vi "close vi.vi"(8 "error in":errorcluster, 11 "vi id":string) -> (0 "error out":errorcluster)   [LabVIEW 2020]
doc: "Closes a currently open VI frontpanel window. If VI was not saved it will be deleted by this."
uses:
  G-AI Core/G-AI Core.lvlib
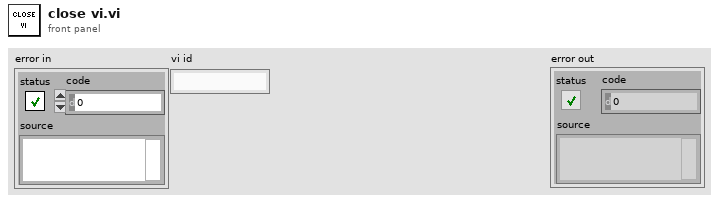
[diagram p1: front panel]
types:
  T1 = enum32{"Invalid", "Standard", "Closed", "Hidden", "Minimized", "Maximized"}
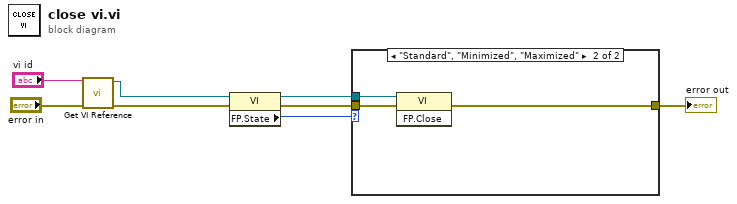
[diagram p0: block diagram]
diagram:
  n1 = call "Get VI Reference.vi"("error in"="error in", "id"="vi id") -> ("error out"=w6:errorcluster, "vi reference"=w3:refnum<vi>)  [unwired: 8 in]
  n2 = property class="VI"(reference=w3, error in=w6) -> (reference out=w2:refnum<vi>, error out=w4:errorcluster, "FP.State"=w1:T1)
  n3 = case shown="\"Standard\", \"Minimized\", \"Maximized\"" w1 {
    tunnel: [w9 w12] -> w5
    tunnel: w4 -> [w9 w11]
    tunnel: w2 -> [_ w10]
    frame Default {
    }
    frame "Standard", "Minimized", "Maximized" {
      n4 = invoke class="VI" method="FP.Close"(reference=w10, error in=w11) -> (error out=w12:errorcluster)  [unwired: 1 in, 2 out]
    }
  }
  "error out" <- w5
